vi "myRIO v1.0 AudioOut Block Write.vi"(5 "Wait Until Done?":bool, 6 "AudioOut FIFO Sample Rate":dbl=1000.0 min=1000.0 max=80000.0, 7 "Scale Constants Array":T1, 8 "error in (no error)":errorcluster, 9 "dbl Scaled Value List":dbl[][](array[numeric]), 10 "AudioOut (N Samples) Channel List":T5, 11 "myRIO Ref In":T3) -> (0 "error out":errorcluster, 3 "myRIO Ref Out":T3)   [LabVIEW 2021]
uses:
  <vilib>/myRIO/Common/Instrument Driver Framework/myRIO v1.0/AudioOut Block/typedefs/AudioOut Block Channels List.ctl
  <vilib>/myRIO/Common/Instrument Driver Framework/myRIO v1.0/AudioOut Block/typedefs/AudioOut Block Channels Enum.ctl
  <vilib>/myRIO/Common/Instrument Driver Framework/Utilities/typedefs/myRIO v1.0 Reference.ctl
  <vilib>/myRIO/Common/Instrument Driver Framework/Utilities/typedefs/Generic FPGA Reference.ctl
  <vilib>/myRIO/Common/Instrument Driver Framework/Utilities/typedefs/Analog Scaling Constants List.ctl
  <vilib>/myRIO/Common/Instrument Driver Framework/Utilities/typedefs/Analog Scaling Constants.ctl
  <vilib>/myRIO/Common/Instrument Driver Framework/myRIO v1.0/AudioOut Block/typedefs/AudioOut Block Channels FPGA Reference.ctl
  <vilib>/myRIO/Common/Instrument Driver Framework/myRIO v1.0/AudioOut Block/typedefs/AudioOut Block Configuration.ctl
  <vilib>/myRIO/Common/Instrument Driver Framework/myRIO v1.0/Resource Manager/vis/myRIO v1.0 Block Write Configuration.vi
  <vilib>/rvi/errors/niLvFpgaAdjustHostInterfaceError.vi
  <vilib>/RVI Host/nirviSupport.llb/nirviErrorClusterFromErrorCode.vi
  <vilib>/rvi/interface/nirviReadWriteControl/nirviReadWriteControl.xnode
  <vilib>/rvi/interface/nirviMethod/nirviMethod.xnode
  <vilib>/rvi/interface/Simulation/niFpgaSimulationCallBeginRW.vi
  <vilib>/rvi/interface/nirviMethod/StockFPGA_InlinedMethodWaitForSingleIRQ.vi
  <vilib>/FPGAPlugInAG/Dynamic/niLvFpga_WaitOnIrq_Dynamic.vi
  <vilib>/FPGAPlugInAG/Dynamic/niLvFpga_AcknowledgeIrq_Dynamic.vi
  NiFpgaLv.dll
  <vilib>/FPGAPlugInAG/Dynamic/niLvFpga_WriteFifo_Dynamic.vi
  <vilib>/rvi/errors/niLvFpgaMergeErrorWithErrorCode.vi
panel:
  # "This VI writes audio values to user specified audio output channels on the myRIO v1.0 hardware. The values are input as dbl values and scaled to u16 for input to the FPGA based on the specifications of the DAC. Please see Block Diagram for details."
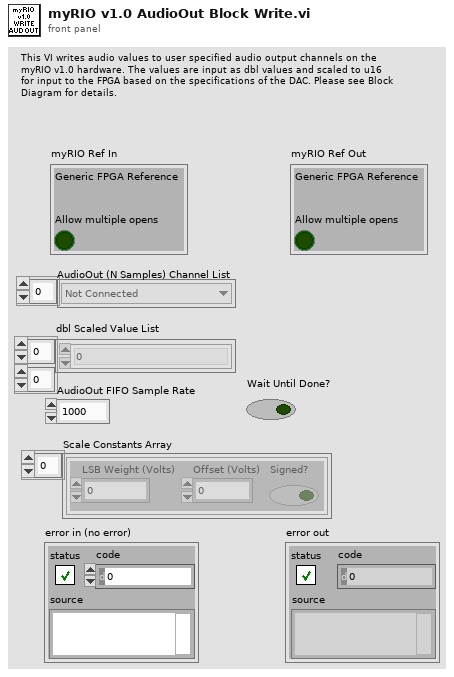
[diagram p1: front panel]
types:
  T1 = typedef "Analog Scaling Constants List.ctl" = T2[]
  T2 = typedef "Analog Scaling Constants.ctl" = cluster{"LSB Weight (Volts)":dbl, "Offset (Volts)":dbl, "Signed?":bool}
  T3 = typedef "myRIO v1.0 Reference.ctl" = cluster{"Generic FPGA Reference":T4, "Allow multiple opens":bool}
  T4 = typedef "Generic FPGA Reference.ctl" = refnum<k20>
  T5 = typedef "AudioOut Block Channels List.ctl" = T6[]
  T6 = typedef "AudioOut Block Channels Enum.ctl" = enum16{"Not Connected", "AudioOut/Left (N Samples)", "AudioOut/Right (N Samples)"}
  T7 = typedef "AudioOut Block Channels FPGA Reference.ctl" = refnum<k20>
  T8 = typedef "AudioOut Block Configuration.ctl" = cluster{"Wait Until Done?":bool, "AudioOut FIFO Sample Rate(ticks)":u32, "Occurrence Handler":refnum<k4>, "Audio data reference":refnum<data-value>}
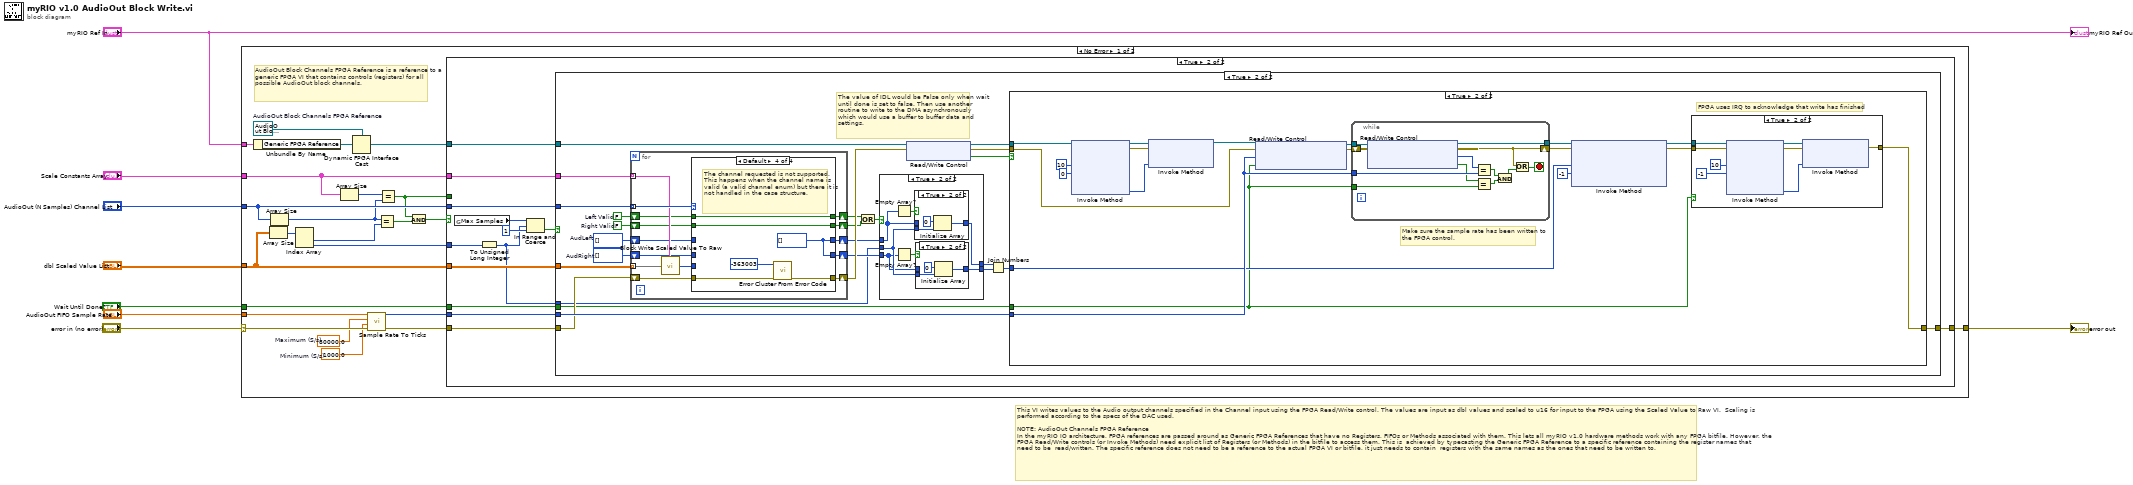
[diagram p0: block diagram]
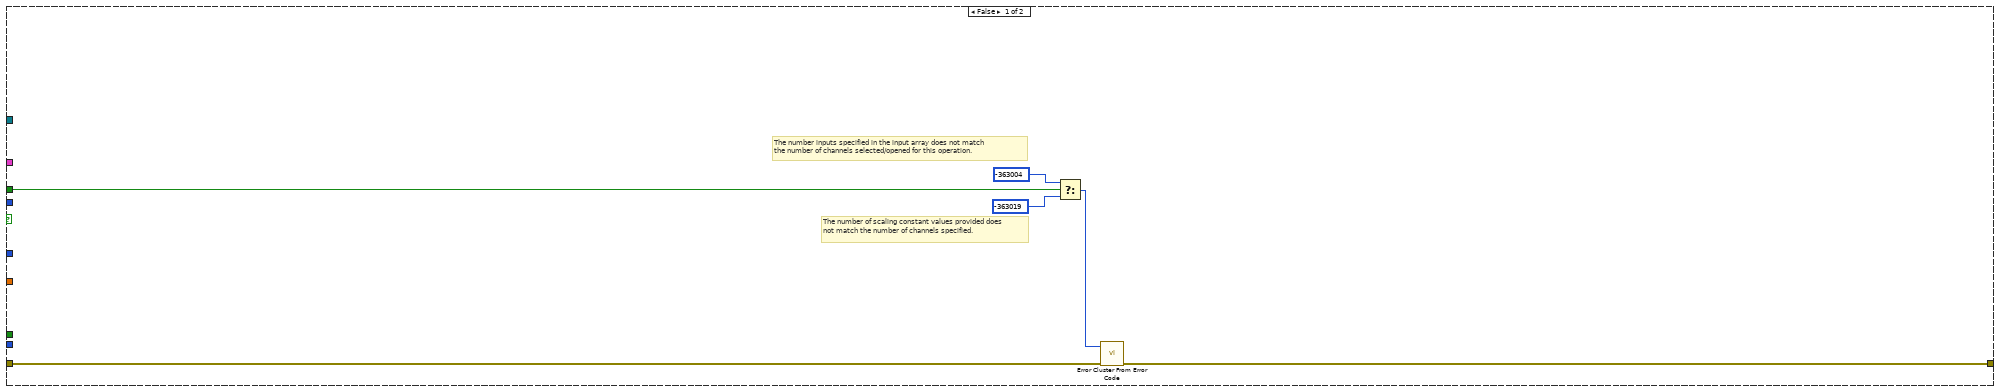
[diagram p2: hidden frame]
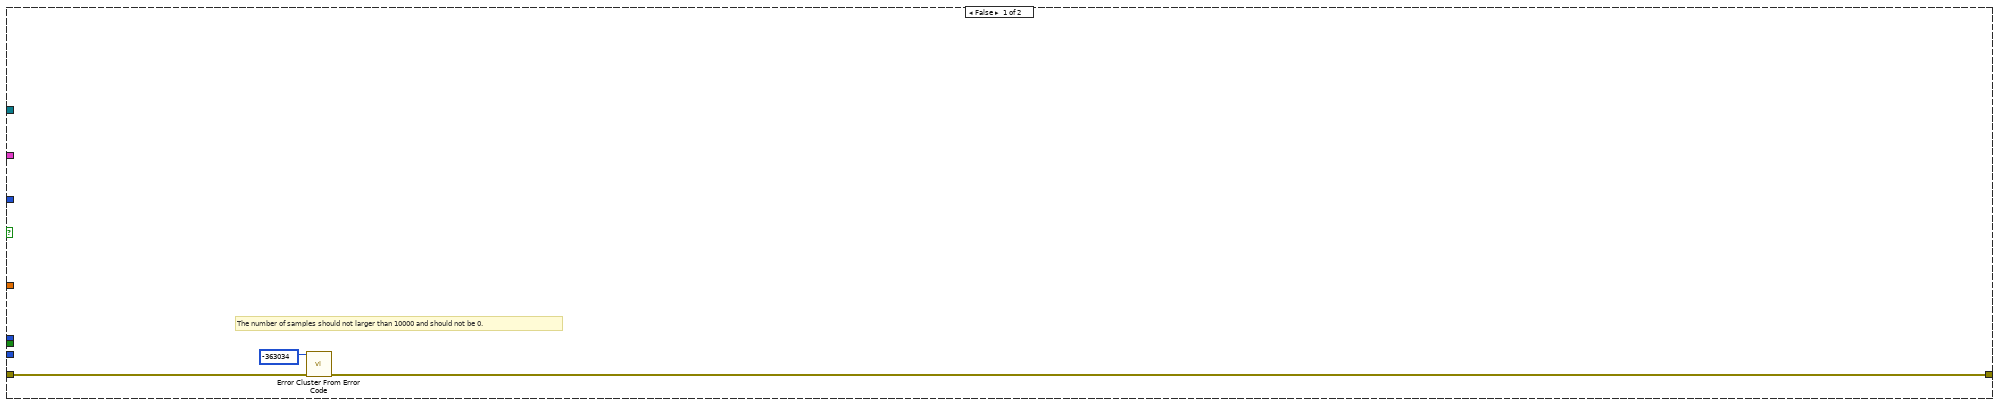
[diagram p3: hidden frame]
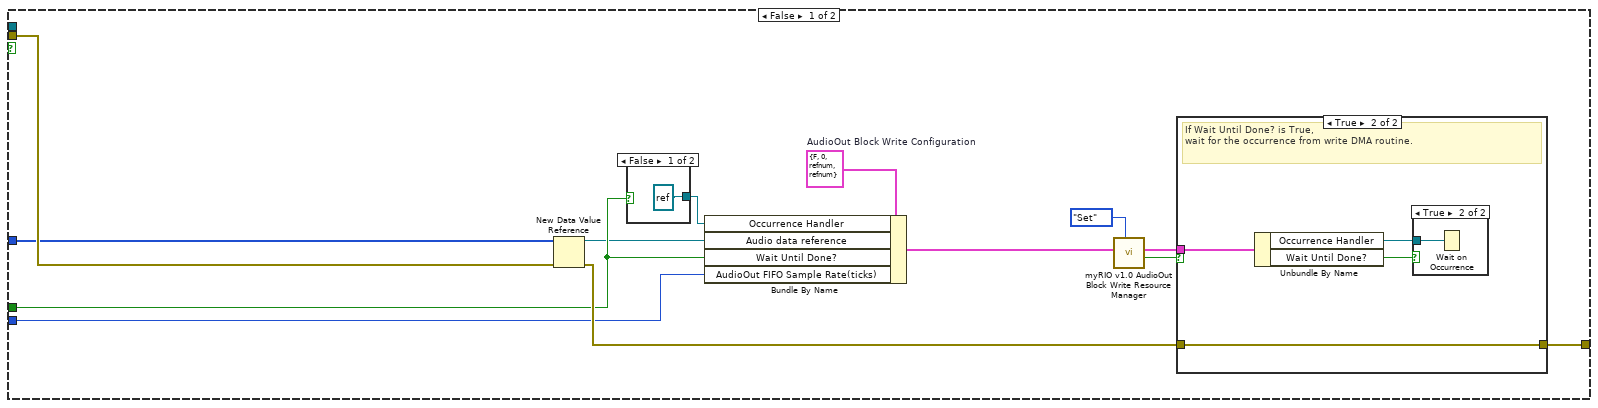
[diagram p7: hidden frame]
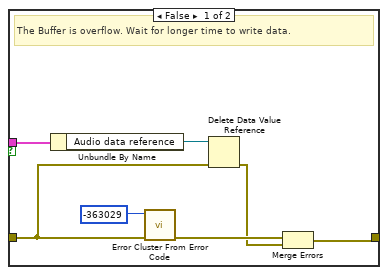
[diagram p8: hidden frame]
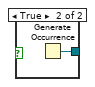
[diagram p10: hidden frame]
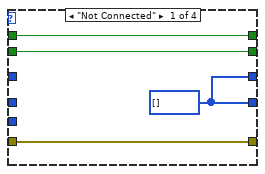
[diagram p12: hidden frame]
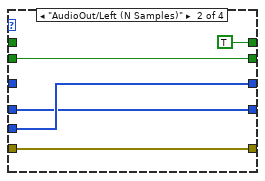
[diagram p13: hidden frame]
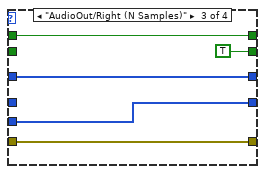
[diagram p14: hidden frame]
diagram:
  # "This VI writes values to the Audio output channels specified in the Channel input using the FPGA Read/Write control. The values are input as dbl values and scaled to u16 for input to the FPGA using the Scaled Value to Raw VI.  Scaling is performed according to the specs of the DAC used.\n\nNOTE: AudioOut Channels FPGA Reference\nIn the myRIO IO architecture, FPGA references are passed around as Generic FPGA References that have no Registers, FIFOs or Methods associated with them. This lets all myRIO v1.0 hardware methods work with any FPGA bitfile. However, the  FPGA Read/Write controls (or Invoke Methods) need explicit list of Registers (or Methods) in the bitfile to access them. This is  achieved by typecasting the Generic FPGA Reference to a specific reference containing the register names that need to be  read/written. The specific reference does not need to be a reference to the actual FPGA VI or bitfile, it just needs to contain  registers with the same names as the ones that need to be written to."
  n1 = case shown="No Error" "error in (no error)" {
    selector: "error in (no error)" -> [w11 w197]
    tunnel: [w31 w197] -> w8
    tunnel: "AudioOut (N Samples) Channel List" -> [w30 _]
    tunnel: "dbl Scaled Value List" -> [w29 _]
    tunnel: "myRIO Ref In" -> [w28 _]
    tunnel: "AudioOut FIFO Sample Rate" -> [w12 _]
    tunnel: "Scale Constants Array" -> [w21 _]
    tunnel: "Wait Until Done?" -> [w15 _]
    frame No Error {
      w9 = 1000.0  # Minimum (S/s)
      w10 = 80000.0  # Maximum (S/s)
      w18 = T7 refnum  # AudioOut Block Channels FPGA Reference
      # "AudioOut Block Channels FPGA Reference is a reference to a generic FPGA VI that contains controls (registers) for all possible AudioOut block channels."
      n2 = Unbundle By Name(w28) -> ("Generic FPGA Reference"=w17:T4)
      n3 = Array Size(array=w29) -> (size(s)=w27:i32[])
      n4 = Array Size(array=w30) -> (size(s)=w25:i32)
      n5 = Index Array(array=w27) -> (element #1=w20:i32, element #2=w19:i32)  [unwired: 2 in]
      n6 = Array Size(array=w21) -> (size(s)=w26:i32)
      n7 = Dynamic FPGA Interface Cast(Session In=w18, Type=w17) -> (Session Out=w16:T7)
      n8 = call <vilib>:"Sample Rate To Ticks.vi"("error in (no error)"=w11, "Minimum (S/s)"=w9, "Maximum (S/s)"=w10, "Sample Rate (S/s)"=w12) -> ("error out"=w13:errorcluster, "Count (tick/s)"=w14:u32)  [unwired: 5 in, 1 out]
      n9 = Equal?(x=w25, y=w20) -> (x = y?=w24:bool)
      n10 = Equal?(x=w26, y=w25) -> (x = y?=w22:bool)
      n11 = And(x=w22, y=w24) -> (x .and. y?=w23:bool)
      n12 = case shown="True" w23 {
        tunnel: w13 -> [w37 w45]
        tunnel: w16 -> [_ w44]
        tunnel: [w36 w48] -> w31
        tunnel: w30 -> [_ w50]
        tunnel: w29 -> [_ w49]
        tunnel: w14 -> [_ w46]
        tunnel: w22 -> [w32 _]
        tunnel: w21 -> [_ w47]
        tunnel: w19 -> [_ w43]
        tunnel: w15 -> [_ w42]
        frame False {
          # "The number of scaling constant values provided does not match the number of channels specified."
          # "The number inputs specified in the input array does not match\nthe number of channels selected/opened for this operation."
          n13 = Select(t=-363004 ("error code (0)"), s=w32, f=-363019 ("error code (0)")) -> (s? t:f=w33:i32)
          n14 = call <vilib>:"Error Cluster From Error Code.vi"("error in (no error)"=w37, "error code (0)"=w33) -> ("error out"=w36:errorcluster)  [unwired: 7 in]
        }
        frame True {
          n15 = global read "myRIO v1.0 Block Write Configuration.vi" "Max Samples"() -> (w41:u32)
          n16 = To Unsigned Long Integer(number=w43) -> (unsigned 32bit integer=w39:u32)
          n17 = In Range and Coerce(upper limit=w41, x=w39, lower limit=u32 1) -> (In Range?=w38:bool)  [unwired: 1 out]
          n18 = case shown="True" w38 {
            tunnel: w50 -> [_ w78]
            tunnel: w49 -> [_ w77]
            tunnel: [w51 w75] -> w48
            tunnel: w47 -> [_ w74]
            tunnel: w46 -> [_ w73]
            tunnel: w45 -> [w52 w72]
            tunnel: w44 -> [_ w66]
            tunnel: w39 -> [_ w54]
            tunnel: w42 -> [_ w71]
            frame False {
              # "The number of samples should not larger than 10000 and should not be 0."
              n19 = call <vilib>:"Error Cluster From Error Code.vi"("error in (no error)"=w52, "error code (0)"=-363034) -> ("error out"=w51:errorcluster)  [unwired: 7 in]
            }
            frame True {
              w62 = u16[] []  # AudRight
              w63 = u16[] []  # AudLeft
              w64 = FALSE  # Right Valid
              w65 = FALSE  # Left Valid
              # "The value of IDL would be False only when wait until done is set to false. Then use another routine to write to the DMA asynchronously which would use a buffer to buffer data and settings."
              n20 = for {
                tunnel: w77 -> [w174] mode=indexing
                tunnel: w78 -> [w172] mode=indexing
                shift-right: [w175] -> w76
                shift-left: w72 -> [w176]
                tunnel: w74 -> [w171] mode=indexing
                shift-right: [w166] -> w56
                shift-left: w65 -> [w170]
                shift-right: [w165] -> w55
                shift-left: w64 -> [w167]
                shift-right: [w169] -> w61
                shift-left: w63 -> [w163]
                shift-right: [w168] -> w60
                shift-left: w62 -> [w164]
                n21 = call <vilib>:"Block Write Scaled Value To Raw.vi"("Scaling Constants"=w171, "dbl Scaled Value"=w174) -> ("u16 Raw Value"=w173:u16[])  [unwired: 7 in]
                n22 = case shown="Default" w172 {
                  tunnel: w176 -> [w180 w185 w190 w194]
                  tunnel: [w180 w185 w190 w195] -> w175
                  tunnel: w173 -> [_ w184 w189 _]
                  tunnel: w170 -> [w178 _ w188 w192]
                  tunnel: [w179 w184 w186 w193] -> w169
                  tunnel: [w179 w181 w189 w193] -> w168
                  tunnel: w167 -> [w177 w182 _ w191]
                  tunnel: [w178 TRUE ("Left Valid") w188 w192] -> w166
                  tunnel: [w177 w182 TRUE ("Right Valid") w191] -> w165
                  tunnel: w164 -> [_ w181 _ _]
                  tunnel: w163 -> [_ _ w186 _]
                  frame "Not Connected" {
                    w179 = u16[] [] ("u16 Raw Value")
                  }
                  frame "AudioOut/Left (N Samples)" {
                  }
                  frame "AudioOut/Right (N Samples)" {
                  }
                  frame Default {
                    w193 = u16[] [] ("u16 Raw Value")
                    # "The channel requested is not supported. This happens when the channel name is valid (a valid channel enum) but there it is not handled in the case structure."
                    n23 = call <vilib>:"Error Cluster From Error Code.vi"("error in (no error)"=w194, "error code (0)"=-363003) -> ("error out"=w195:errorcluster)  [unwired: 7 in]
                  }
                }
              }
              n24 = Or(x=w56, y=w55) -> (x .or. y?=w57:bool)
              n25 = case shown="True" w57 {
                tunnel: w61 -> [w80 w82]
                tunnel: w60 -> [w79 w81]
                tunnel: [w80 w84] -> w59
                tunnel: [w79 w83] -> w58
                tunnel: w54 -> [_ w85]
                frame False {
                  # "Both Left and Right data\nare invalid."
                }
                frame True {
                  n26 = Empty Array?(array=w82) -> (empty?=w87:bool)
                  n27 = Empty Array?(array=w81) -> (empty?=w86:bool)
                  n28 = case shown="True" w87 {
                    tunnel: [w92 w94] -> w84
                    tunnel: w85 -> [_ w93]
                    tunnel: w82 -> [w92 _]
                    frame False {
                    }
                    frame True {
                      n29 = Initialize Array ("AudLeft")(u16 0 ("Numeric"), w93) -> (w94:u16[])
                    }
                  }
                  n30 = case shown="True" w86 {
                    tunnel: [w88 w90] -> w83
                    tunnel: w85 -> [_ w89]
                    tunnel: w81 -> [w88 _]
                    frame False {
                    }
                    frame True {
                      n31 = Initialize Array ("AudRight")(u16 0 ("Numeric"), w89) -> (w90:u16[])
                    }
                  }
                }
              }
              n32 = xnode "Read/Write Control"("FPGA VI Reference In"=w66, "error in"=w76) -> ("FPGA VI Reference Out"=w69:T7, "error out"=w68:errorcluster, "AO.AudioOut.IDL"=w70:bool)
              n33 = Join Numbers(hi=w59, lo=w58) -> ((hi.lo)=w67:u32[])
              n34 = case shown="True" w70 {
                tunnel: w69 -> [_ w127]
                tunnel: w68 -> [w107 w125]
                tunnel: [w103 w133] -> w75
                tunnel: w73 -> [w106 w139]
                tunnel: w67 -> [w104 w124]
                tunnel: w71 -> [w105 w123]
                frame False {
                  w100 = T8 {"Wait Until Done?"=FALSE, "AudioOut FIFO Sample Rate(ticks)"=0, "Occurrence Handler"=refnum, "Audio data reference"=refnum}  # AudioOut Block Write Configuration
                  n35 = New Data Value Reference(data value=w104, error in=w107) -> (data value reference=w101:refnum<data-value>, error out=w108:errorcluster)
                  n36 = case shown="False" w105 {
                    tunnel: [refnum<k4> refnum ("occurrence") w122] -> w102
                    frame False {
                    }
                    frame True {
                      n37 = Generate Occurrence() -> (w122:refnum<k4>)
                    }
                  }
                  n38 = Bundle By Name(cluster=w100, "Occurrence Handler"=w102, "Audio data reference"=w101, "Wait Until Done?"=w105, "AudioOut FIFO Sample Rate(ticks)"=w106) -> (w97:T8)
                  n39 = call <vilib>:"myRIO v1.0 AudioOut Block Write Resource Manager.vi"("Action"=enum16{"Get", "Set"}."Set", "AudioOut Resource In"=w97) -> ("Action Succeeds"=w98:bool, "AudioOut Resource Out"=w96:T8)  [unwired: 8 in]
                  n40 = case shown="True" w98 {
                    tunnel: w108 -> [w112 w119]
                    tunnel: [w109 w119] -> w103
                    tunnel: w96 -> [w114 w116]
                    frame False {
                      # "The Buffer is overflow. Wait for longer time to write data."
                      n41 = Unbundle By Name(w114) -> ("Audio data reference"=w113:refnum<data-value>)
                      n42 = call <vilib>:"Error Cluster From Error Code.vi"("error in (no error)"=w112, "error code (0)"=-363029) -> ("error out"=w111:errorcluster)  [unwired: 7 in]
                      n43 = Delete Data Value Reference(data value reference=w113, error in=w112) -> (error out=w110:errorcluster)  [unwired: 1 out]
                      n44 = Merge Errors(w111, w110) -> (w109:errorcluster)
                    }
                    frame True {
                      # "If Wait Until Done? is True, \nwait for the occurrence from write DMA routine."
                      n45 = Unbundle By Name(w116) -> ("Occurrence Handler"=w117:refnum<k4>, "Wait Until Done?"=w118:bool)
                      n46 = case shown="True" w118 {
                        tunnel: w117 -> [_ w120]
                        frame False {
                        }
                        frame True {
                          n47 = Wait on Occurrence(2:w120) -> ()  [unwired: 2 in, 1 out]
                        }
                      }
                    }
                  }
                }
                frame True {
                  # "Make sure the sample rate has been written to the FPGA control."
                  # "FPGA uses IRQ to acknowledge that write has finished"
                  n48 = xnode "Invoke Method"("FPGA VI Reference In"=w127, "IRQ Number(s)"=10, "Timeout (ms)"=0) -> ("FPGA VI Reference Out"=w130:T7, "error out"=w129:errorcluster, "IRQ(s) Asserted"=w128:i32)  [unwired: 1 in, 1 out]
                  n49 = xnode "Invoke Method"("FPGA VI Reference In"=w130, "error in"=w129, "IRQ Number(s)"=w128) -> ("FPGA VI Reference Out"=w126:T7)  [unwired: 1 out]
                  n50 = xnode "Read/Write Control"("FPGA VI Reference In"=w126, "error in"=w125, "AO.AudioOut.SampleRate"=w139, "AO.AudioOut.IRQ.SELECT"=w123) -> ("FPGA VI Reference Out"=w141:T7, "error out"=w140:errorcluster)
                  n51 = while {
                    tunnel: w141 -> [w162]
                    tunnel: [w161] -> w138
                    shift-right: [w157] -> w137
                    shift-left: w140 -> [w160]
                    tunnel: w139 -> [w158]
                    tunnel: w123 -> [w154]
                    stop <- w156 stop-if-true
                    n52 = xnode "Read/Write Control"("FPGA VI Reference In"=w162, "error in"=w160) -> ("FPGA VI Reference Out"=w161:T7, "error out"=w157:errorcluster, "AO.AudioOut.SampleRate"=w159:u32, "AO.AudioOut.IRQ.SELECT"=w155:bool)
                    n53 = Equal?(x=w159, y=w158) -> (x = y?=w152:bool)
                    n54 = Equal?(x=w155, y=w154) -> (x = y?=w153:bool)
                    n55 = And(x=w152, y=w153) -> (x .and. y?=w151:bool)
                    n56 = Or(x=w157, y=w151) -> (x .or. y?=w156:bool)
                  }
                  n57 = xnode "Invoke Method"("FPGA VI Reference In"=w138, "error in"=w137, "Data"=w124, "Timeout (ms)"=-1) -> ("FPGA VI Reference Out"=w135:T7, "error out"=w134:errorcluster)  [unwired: 1 out]
                  n58 = case shown="True" w123 {
                    tunnel: w135 -> [_ w149]
                    tunnel: w134 -> [w142 w148]
                    tunnel: [w142 w144] -> w133
                    frame False {
                    }
                    frame True {
                      n59 = xnode "Invoke Method"("FPGA VI Reference In"=w149, "error in"=w148, "IRQ Number(s)"=10, "Timeout (ms)"=-1) -> ("FPGA VI Reference Out"=w147:T7, "error out"=w146:errorcluster, "IRQ(s) Asserted"=w145:i32)  [unwired: 1 out]
                      n60 = xnode "Invoke Method"("FPGA VI Reference In"=w147, "error in"=w146, "IRQ Number(s)"=w145) -> ("error out"=w144:errorcluster)  [unwired: 1 out]
                    }
                  }
                }
              }
            }
          }
        }
      }
    }
    frame Error {
      # "There is an incoming error so there is nothing to do."
    }
  }
  "error out" <- w8
  "myRIO Ref Out" <- "myRIO Ref In"
